vi "Initialize State Machine.vi"(7 "Input Paths Refnum":refnum<vi>, 8 "error in (no error)":errorcluster, 9 "Bus Info":T1[](array[typedef]), 10 "ProgressBar in":refnum<k24>(container), 11 "Enum Refnum":refnum<vi>) -> (0 "error out":errorcluster, 1 "queue out":refnum<queue>, 2 "ProgressBar out":refnum<k24>, 3 "Notifier out":refnum<notifier>, 5 "Status Log":refnum<file>)   [LabVIEW 2014, in "Initialization and IO Node Scripting.lvlib"]
uses:
  Initialization and IO Node Scripting.lvlib
  System.Windows.Forms
  Scripting States.ctl
  Controls/Bus Information.ctl
  Controls/Device Information.ctl
  Controls/Pin Information.ctl
  Controls/Input Paths.ctl
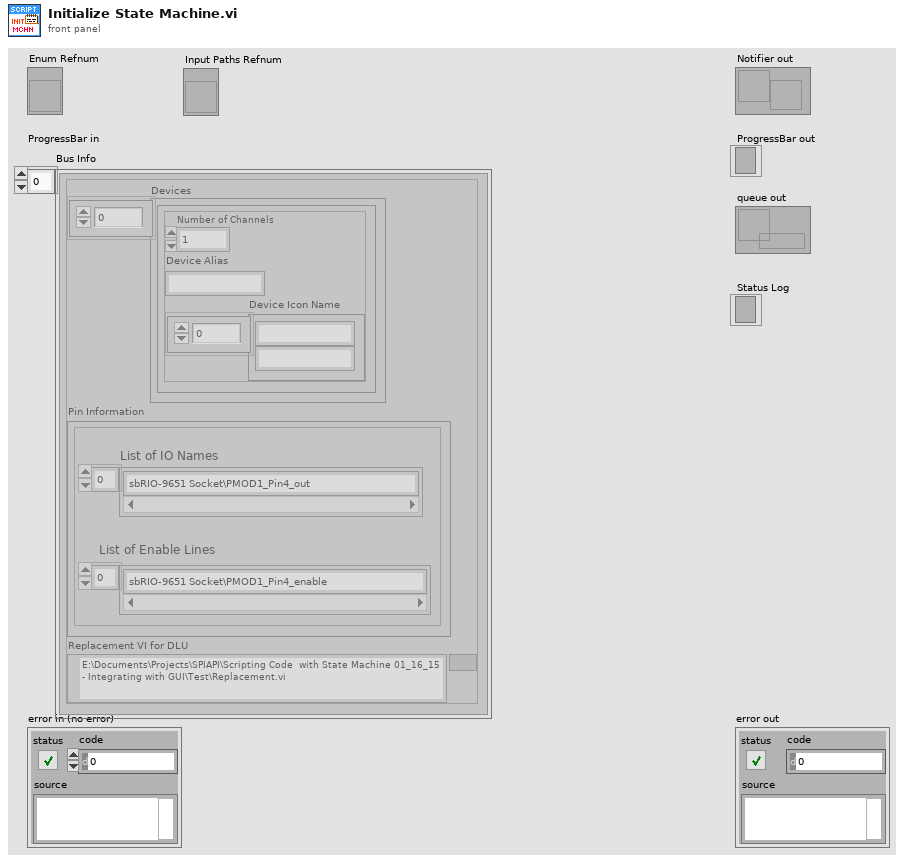
[diagram p1: front panel]
types:
  T1 = typedef "Initialization and IO Node Scripting.lvlib/Bus Information.ctl" = cluster{"Devices":T2[], "Pin Information":T3, "Replacement VI for DLU":path}
  T2 = typedef "Device Information.ctl" = cluster{"Number of Channels":i32, "Device Alias":string, "Device Icon Name":string[]}
  T3 = typedef "Pin Information.ctl" = cluster{"List of IO Names":string[], "List of Enable Lines":string[]}
  T4 = enum16{"open", "replace", "create", "open or create", "replace or create", "replace or create with confirmation"}
  T5 = typedef "Scripting States.ctl" = enum16{"Initialize", "Modify Dequeue Commands", "Modify Enqueue Data", "Create Project FIFOs", "Create and Place IO Nodes", "Update Node Count in Engine", "Expand FIFO Type Def", "Populate FIFO Names in Engine", "Modify I/O Pin Names", "Modify I/O Pin Enable", "Replace DLU", "Place SPI Engine", "Buses Complete Check", "End"}
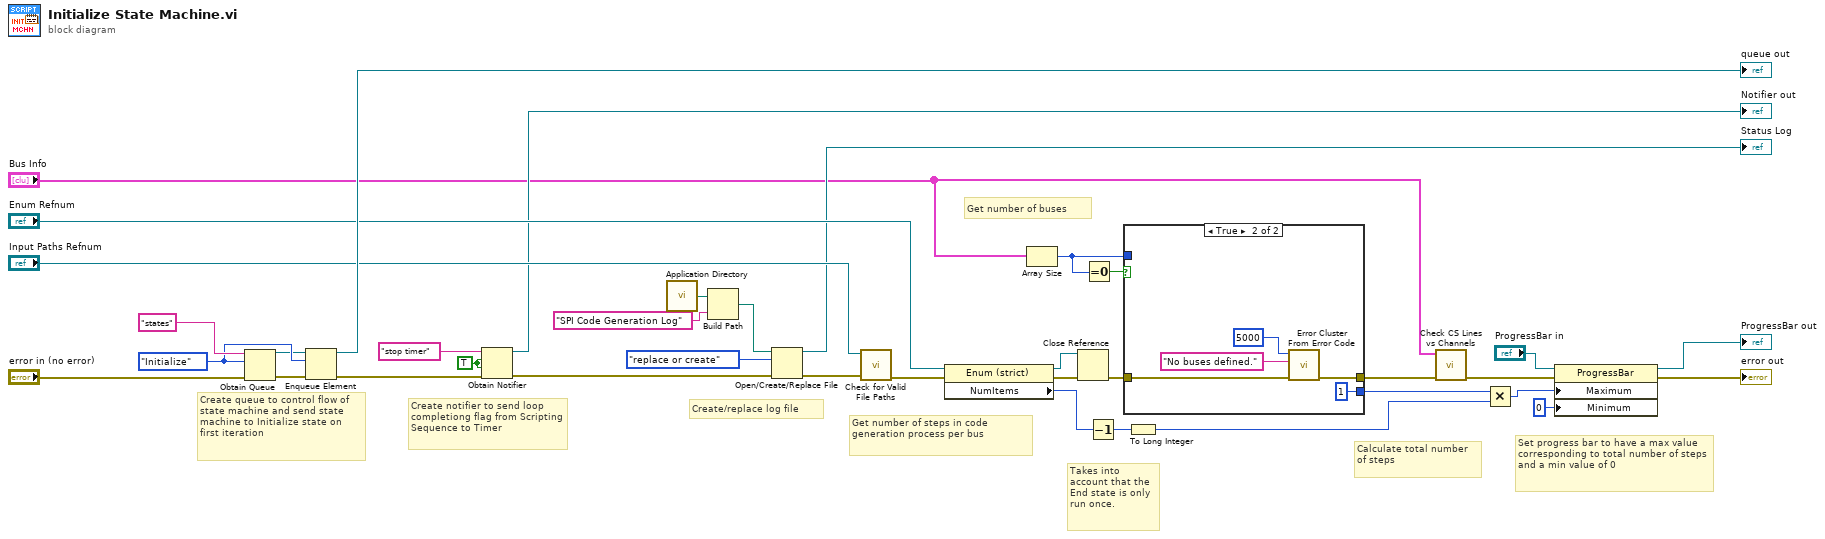
[diagram p0: block diagram]
diagram:
  w16 = TRUE ("create if not found? (T)")
  w30 = Scripting_States."Initialize"
  # "Create/replace log file"
  # "Takes into account that the End state is only run once."
  # "Set progress bar to have a max value corresponding to total number of steps and a min value of 0"
  # "Calculate total number of steps"
  # "Get number of buses"
  # "Get number of steps in code generation process per bus"
  # "Create notifier to send loop completiong flag from Scripting Sequence to Timer"
  # "Create queue to control flow of state machine and send state machine to Initialize state on first iteration"
  n1 = Obtain Queue(name (unnamed)="states", element data type=w30, error in (no error)="error in (no error)") -> (queue out=w29:refnum<queue>, error out=w28:errorcluster)  [unwired: 2 in, 1 out]
  n2 = Enqueue Element(queue=w29, element=w30, error in (no error)=w28) -> (queue out=→"queue out":refnum<queue>, error out=w14:errorcluster)  [unwired: 1 in, 1 out]
  n3 = Obtain Notifier(name (unnamed)="stop timer", notification data type=w16, create if not found? (T)=w16, error in (no error)=w14) -> (notifier out=→"Notifier out":refnum<notifier>, error out=w7:errorcluster)  [unwired: 1 out]
  n4 = call <vilib>:"Application Directory.vi"() -> ("Application Directory"=w9:path)
  n5 = Build Path(base path=w9, name or relative path="SPI Code Generation Log") -> (appended path=w11:path)
  n6 = Open/Create/Replace File(file path (use dialog)=w11, error in=w7, operation (0:open)=T4."replace or create") -> (refnum out=→"Status Log":refnum<file>, error out=w2:errorcluster)  [unwired: 3 in, 1 out]
  n7 = call "Check for Valid File Paths.vi"("error in (no error)"=w2, "Input Paths Refnum"="Input Paths Refnum") -> ("error out"=w18:errorcluster)  [unwired: 9 in]
  n8 = property on="Property Node" class="Enum (strict)"(reference="Enum Refnum", error in=w18) -> (reference out=w34:refnum<vi>, error out=w33:errorcluster, "NumItems"=w26:u32)
  n9 = Array Size(array="Bus Info") -> (size(s)=w19:i32)
  n10 = Close Reference(reference=w34, error in (no error)=w33) -> (error out=w24:errorcluster)
  n11 = Equal To 0?(x=w19) -> (x = 0?=w23:bool)
  n12 = Decrement(x=w26) -> (x-1=w25:u32)
  n13 = case shown="True" w23 {
    tunnel: w24 -> [w39 w44]
    tunnel: [w39 w43] -> w6
    tunnel: [w38 1] -> w22
    tunnel: w19 -> [w38 _]
    frame False {
    }
    frame True {
      n14 = call <vilib>:"Error Cluster From Error Code.vi"("error in (no error)"=w44, "error message (\"\")"="No buses defined." ("error message (\"\")"), "error code (0)"=5000) -> ("error out"=w43:errorcluster)  [unwired: 6 in]
    }
  }
  n15 = To Long Integer(number=w25) -> (32bit integer=w21:i32)
  n16 = call "Check CS Lines vs Channels.vi"("error in"=w6, "Bus Info"="Bus Info") -> ("error out"=w5:errorcluster)  [unwired: 9 in]
  n17 = Multiply(x=w22, y=w21) -> (x*y=w20:i32)
  n18 = property class="ProgressBar"(reference="ProgressBar in", error in=w5, "Maximum"=w20, "Minimum"=0) -> (reference out=→"ProgressBar out":refnum<k24>, error out=→"error out":errorcluster)
